vi "ViresVTD.vi"(10 "Parameters":variant, 11 "Process":refnum<class "Process.lvclass">) -> ()   [LabVIEW 2020, in "Vires VTD Engine.lvlib"]
uses:
  Vires VTD Engine.lvlib
  <vilib>/NI/NIVS Inline Async API/_VS Inline Async API/Process/Process.lvclass
  Type/Status_Cluster.ctl
  Type/ConnectionStatus.ctl
  Type/CaseSelection.ctl
  Shared/Compiled.Settings.ctl
  System Explorer/RDB Data.ctl
  RDB/RDB Object.ctl
  RDB/RDB Player Object.ctl
  Shared/Network Settings.ctl
  Shared/Protocol.ctl
  Shared/SensorInfos.ctl
  Shared/SensorInfo.ctl
  Shared/Sensor Name.ctl
  MM/MM Data.ctl
  MM/MM Objects.ctl
  MM/MM Object.ctl
  <vilib>/NI/NIVS Inline Async API/_VS Inline Async API/Process/Process.lvclass/Process.ctl
  <vilib>/NI/NIVS Inline Async API/_Data Access Engine/Access Type Classes/Write/Write.lvclass/Write.ctl
  <vilib>/NI/NIVS Inline Async API/_Data Access Engine/Access Type Classes/Read/Read.lvclass/Read.ctl
  <vilib>/NI/NIVS Inline Async API/_Data Access Engine/Data Access Engine/Methods/Write.Data.vi
  <vilib>/NI/NIVS Inline Async API/_Data Access Engine/Data Access Engine/Methods/Read.Data.vi
  <vilib>/NI/NIVS Inline Async API/_VS Inline Async API/Process/Data Member Access/Read Data Access.vi
  <vilib>/NI/NIVS Inline Async API/_VS Inline Async API/Error Handling Process/SubVIs/Error.ConvertArray.vi
  <vilib>/NI/NIVS Inline Async API/_Data Access Engine/Access Type Classes/Write/Write.ProcessData.vi
  <vilib>/NI/NIVS Inline Async API/_Data Access Engine/Access Type Classes/Read/Read.ProcessData.vi
  <vilib>/NI/NIVS Inline Async API/_Data Access Engine/Access Type Classes/Write/Write.Buffer.vi
  <vilib>/NI/NIVS Inline Async API/_Data Access Engine/Access Type Classes/Write/Write.Commit.vi
  <vilib>/NI/NIVS Inline Async API/_Data Access Engine/Data Access Engine/Methods/ReadWrite.Lookup.vi
  <vilib>/NI/NIVS Inline Async API/_Data Access Engine/Data Access Engine/Methods/Write.Lookup.vi
  <vilib>/NI/NIVS Inline Async API/_Data Access Engine/Data Access Engine/Methods/Read.Lookup.vi
  <vilib>/NI/NIVS Inline Async API/_Data Access Engine/Data Access Engine/Data Access Engine.lvclass
  RDB/RDB.lvlib
  Shared/Vires VTD Shared.lvlib
  MM/MM.lvlib
  SCP/SCP.lvlib
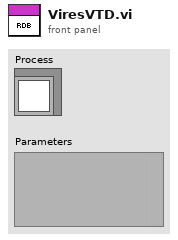
[diagram p1: front panel]
types:
  T1 = typedef "Vires VTD Engine.lvlib/Status_Cluster.ctl" = cluster{"simTime":dbl, "simFrame":dbl, "Connection Status":T2, "Connection Command":enum16{"Disconnect", "Connect"}, "Last Error":i32, "Case selection":T3}
  T2 = typedef "Vires VTD Engine.lvlib/ConnectionStatus.ctl" = enum16{"Disconnected", "Connected"}
  T3 = typedef "Vires VTD Engine.lvlib/CaseSelection.ctl" = enum32{"Idle", "Connecting", "Disconnecting", "Read/Write"}
  T4 = typedef "Vires VTD Shared.lvlib/Compiled.Settings.ctl" = cluster{"Name":string, "RDB Data Receive ":T5, "RDB Data Sent":T5, "vclient":path, "Network Settings":T8, "SensorInfos":T10, "mmanager":path, "Scenario Paths":string[], "Custom SCP Commands":string[]}
  T5 = typedef "Vires VTD Shared.lvlib/RDB Data.ctl" = T6[]
  T6 = typedef "RDB.lvlib/RDB Object.ctl" = cluster{"pkID":i32, "RDB Player Objects":T7[]}
  T7 = typedef "RDB.lvlib/RDB Player Object.ctl" = cluster{"PlayerID":i32, "Signals":string[], "WheelID":i32}
  T8 = typedef "Vires VTD Shared.lvlib/Network Settings.ctl" = cluster{"IP adress":string, "RDB":cluster{"Protocol":T9, "Tx Port":u16, "Rx Port":u16, "Buffer Size":i32, "Timeout":u16}, "SCP":cluster{"Protocol":T9, "Tx Port":u16, "Rx Port":u16, "Buffer Size":i32, "Timeout":u16}}
  T9 = typedef "Vires VTD Shared.lvlib/Protocol.ctl" = enum16{"UDP", "TCP"}
  T10 = typedef "Vires VTD Shared.lvlib/SensorInfos.ctl" = T11[]
  T11 = typedef "Vires VTD Shared.lvlib/SensorInfo.ctl" = cluster{"Sensor Name":T12, "Protocol":T9, "Network port":i32, "# Culled Objects":i32, "PlayerID":u8, "MM Data":T13}
  T12 = typedef "Vires VTD Shared.lvlib/Sensor Name.ctl" = string
  T13 = typedef "Vires VTD Shared.lvlib/MM Data.ctl" = T14[]
  T14 = typedef "MM.lvlib/MM Objects.ctl" = cluster{"pkID":i32, "MM Objects":T15[]}
  T15 = typedef "MM.lvlib/MM Object.ctl" = cluster{"Object":i32, "Signals":string[]}
  T16 = typedef "Data Access Engine.lvlib/Data Access Engine.lvclass/ReadWrite.DVR.ctl" = refnum<data-value>
  T17 = typedef "Data Access Engine.lvlib/Data Access Engine.lvclass/Write.DVR.ctl" = refnum<data-value>
  T18 = typedef "Data Access Engine.lvlib/Data Access Engine.lvclass/Read.DVR.ctl" = refnum<data-value>
  T19 = typedef "RDB.lvlib/RDB References.ctl" = cluster{"RDB Receive Reference":T20, "RDB Send Reference":T20}
  T20 = typedef "RDB.lvlib/RDB Reference.ctl" = cluster{"Conversion References":refnum<k21>[], "RDB Data":T21[], "RDB Signals":dbl[], "noSignals":i32[]}
  T21 = typedef "XNET Frame FlexRay.ctl" = cluster{"timestamp":timestamp, "payload":u8[], "slot":u16, "type":T22, "cycle count":u8, "startup?":bool, "sync?":bool, "preamble?":bool, "ch A":bool, "ch B":bool, "echo?":bool}
  T22 = typedef "XNET Frame Type FlexRay.ctl" = u8
  T23 = typedef "Vires VTD Engine.lvlib/Settings.ctl" = cluster{"UDP Receiver":refnum<k16>, "UDP Sender":refnum<k16>, "Valid Packet":bool, "TCP":refnum<k5>, "Network Settings":T8, "vclient":path}
  T24 = typedef "SCP.lvlib/SCP_Cluster.ctl" = cluster{"SCP Command ":i32, "Custom SCP Command Index":i32, "Simulation Time":i32, "Step Size":i32, "Scenario Selection":i32, "Last SCP Error":i32, "Scenario Paths":string[], "Custom SCP Commands":string[]}
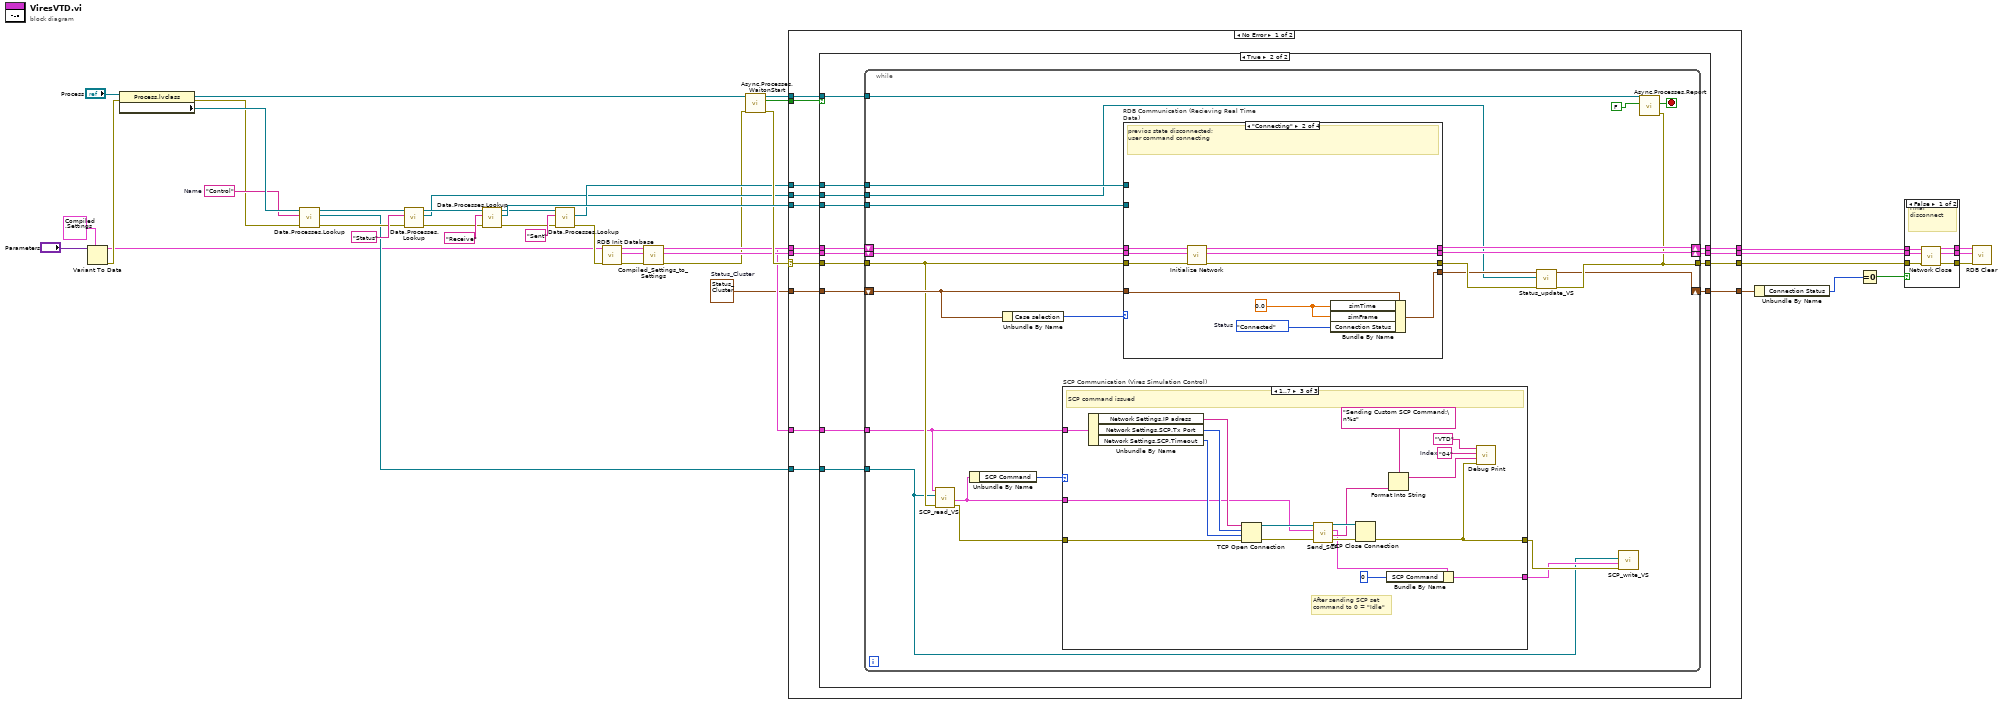
[diagram p0: block diagram]
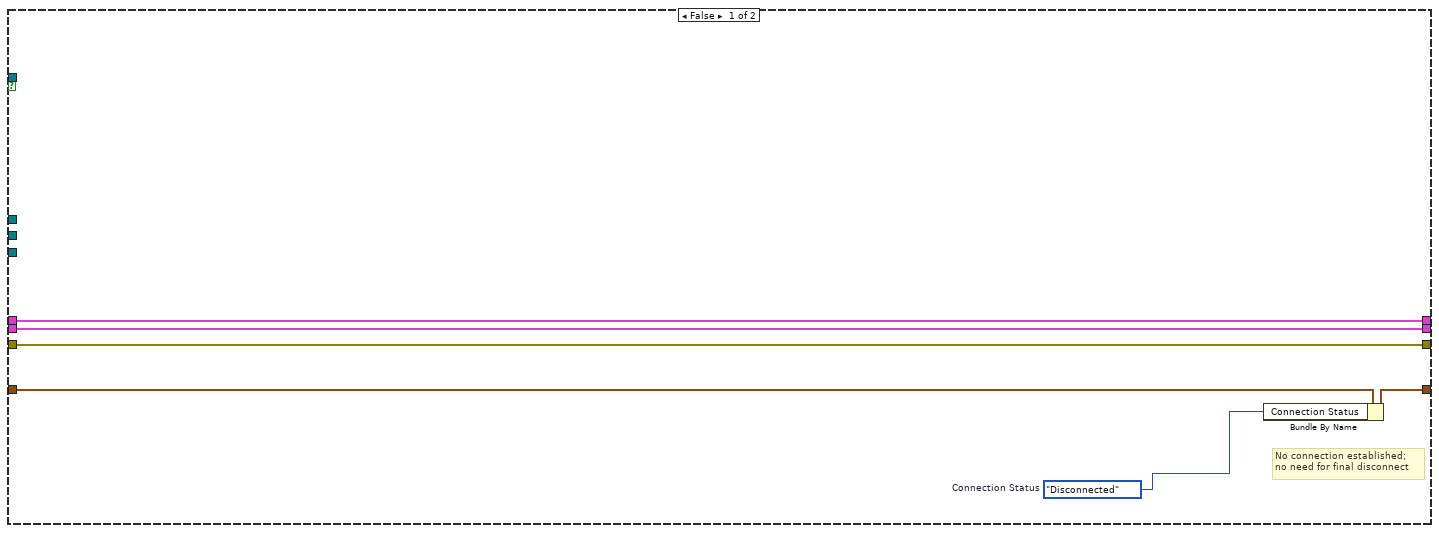
[diagram p2: hidden frame]
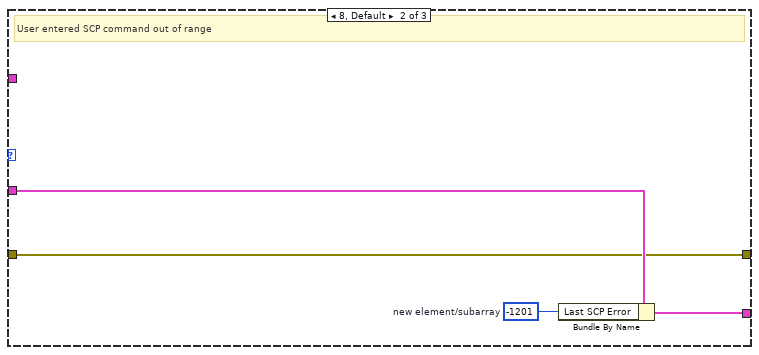
[diagram p4: hidden frame]
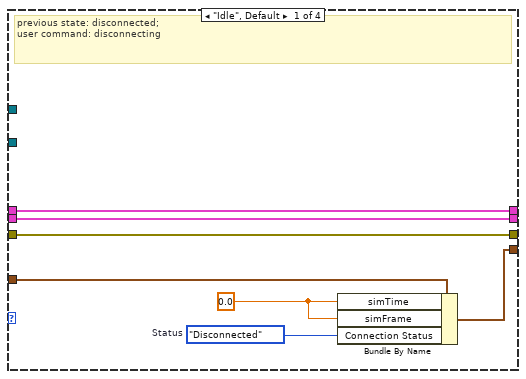
[diagram p5: hidden frame]
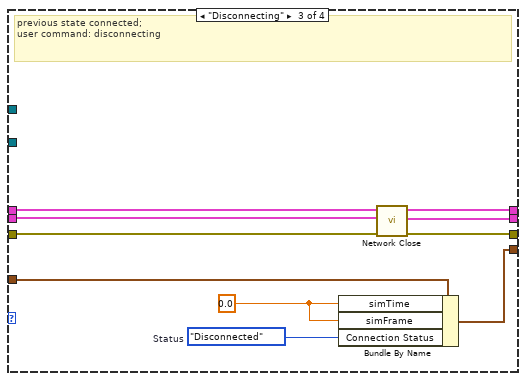
[diagram p6: hidden frame]
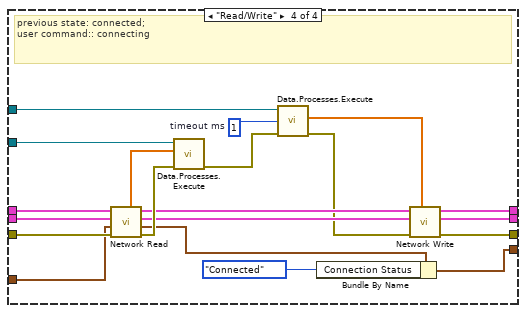
[diagram p7: hidden frame]
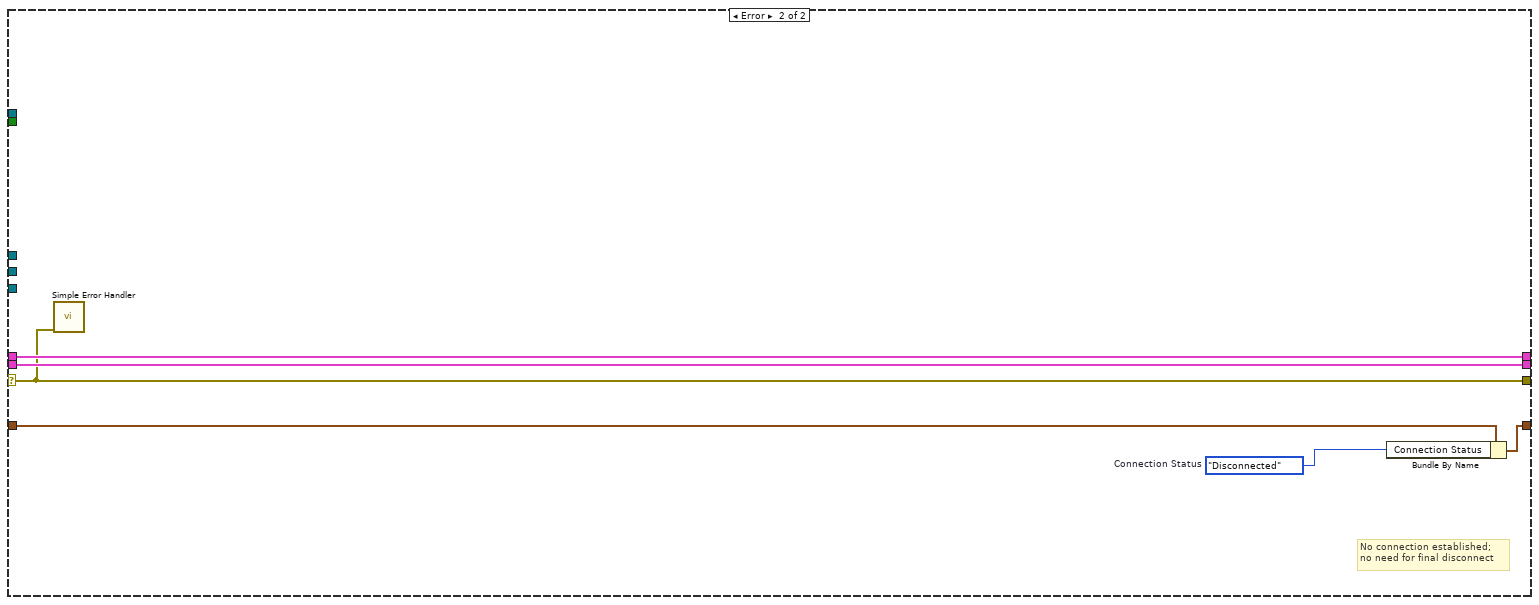
[diagram p8: hidden frame]
diagram:
  w1 = T1 {"simTime"=0.0, "simFrame"=0.0, "Connection Status"=enum."Disconnected", "Connection Command"=enum."Disconnect", "Last Error"=0, "Case selection"=enum."Connecting"}  # Status_Cluster
  w9 = "Control"  # Name
  n1 = Variant To Data(type=T4 {"Name"="", "RDB Data Receive "=[], "RDB Data Sent"=[], "vclient"=path "", "Network Settings"={"IP adress"="127.0.0.1", "RDB"={"Protocol"=enum."TCP", "Tx Port"=10, "Rx Port"=10, "Buffer Size"=204800, "Timeout"=10}, "SCP"={"Protocol"=enum."UDP", "Tx Port"=48190, "Rx Port"=48190, "Buffer Size"=204800, "Timeout"=10}}, "SensorInfos"=[], "mmanager"=path "", "Scenario Paths"=[], "Custom SCP Commands"=[]} ("Compiled.Settings"), Variant="Parameters") -> (data=w6:T4, error out=w24:errorcluster)  [unwired: 1 in]
  n2 = property class="Process.lvclass"(reference="Process", error in=w24) -> (reference out=w33:refnum<class "Process.lvclass">, error out=w7:errorcluster, "Data Member Access:Data Access"=w12:refnum<class "Data Access Engine.lvclass">)
  n3 = call-poly <vilib>:"Data.Processes.Lookup.vi"("error in (no error)"=w7, "Name"=w9, "Data Access API in"=w12) -> ("error out"=w10:errorcluster, "Ref"=w8:T16, "Data Access API out"=w11:refnum<class "Data Access Engine.lvclass">)  [unwired: 5 in, 1 out]
  n4 = call-poly <vilib>:"Data.Processes.Lookup.vi"("error in (no error)"=w10, "Name"="Status" ("Item Name"), "Data Access API in"=w11) -> ("error out"=w28:errorcluster, "Ref"=w25:T16, "Data Access API out"=w27:refnum<class "Data Access Engine.lvclass">)  [unwired: 5 in, 1 out]
  n5 = call-poly <vilib>:"Data.Processes.Lookup.vi"("error in (no error)"=w28, "Name"="Receive", "Data Access API in"=w27) -> ("error out"=w37:errorcluster, "Ref"=w36:T17, "Data Access API out"=w35:refnum<class "Data Access Engine.lvclass">)  [unwired: 5 in, 1 out]
  n6 = call-poly <vilib>:"Data.Processes.Lookup.vi"("error in (no error)"=w37, "Name"="Sent", "Data Access API in"=w35) -> ("error out"=w23:errorcluster, "Ref"=w29:T18)  [unwired: 5 in, 2 out]
  n7 = call "RDB Init Database.vi"("error in"=w23, "Compiled.Settings"=w6) -> ("error out"=w22:errorcluster, "RDB References"=w20:T19, "Compiled.Settings"=w4:T4)  [unwired: 7 in]
  n8 = call "Compiled_Settings_to_Settings.vi"("error in (no error)"=w22, "Compiled.Settings"=w4) -> ("error out"=w5:errorcluster, "Settings"=w21:T23)  [unwired: 8 in]
  n9 = call <vilib>:"Async.Processes.WaitonStart.vi"("error in (no error)"=w5, "Process"=w33) -> ("error out"=w31:errorcluster, "Execute"=w41:bool, "Process out"=w40:refnum<class "Process.lvclass">)  [unwired: 7 in]
  n10 = case shown="No Error" w31 {
    selector: w31 -> [w51 w176]
    tunnel: w41 -> [w56 _]
    tunnel: w40 -> [w55 _]
    tunnel: w36 -> [w54 _]
    tunnel: w21 -> [w53 w178]
    tunnel: w20 -> [w52 w177]
    tunnel: w29 -> [w50 _]
    tunnel: [w49 w178] -> w15
    tunnel: [w48 w177] -> w14
    tunnel: w25 -> [w47 _]
    tunnel: [w46 w176] -> w16
    tunnel: w8 -> [w45 _]
    tunnel: w4 -> [w44 _]
    tunnel: [w43 w175] -> w3
    tunnel: w1 -> [w42 w174]
    frame No Error {
      n11 = case shown="True" w56 {
        tunnel: w51 -> [w60 w67]
        tunnel: w55 -> [_ w69]
        tunnel: w54 -> [_ w76]
        tunnel: w53 -> [w62 w68]
        tunnel: w52 -> [w61 w75]
        tunnel: w50 -> [_ w74]
        tunnel: [w62 w73] -> w49
        tunnel: [w61 w72] -> w48
        tunnel: w47 -> [_ w71]
        tunnel: [w60 w70] -> w46
        tunnel: w45 -> [_ w66]
        tunnel: w44 -> [_ w65]
        tunnel: [w59 w64] -> w43
        tunnel: w42 -> [w58 w63]
        frame False {
          w57 = ConnectionStatus."Disconnected"  # Connection Status
          # "No connection established;\nno need for final disconnect"
          n12 = Bundle By Name(cluster=w58, "Connection Status"=w57) -> (w59:T1)
        }
        frame True {
          n13 = while {
            tunnel: w69 -> [w100]
            tunnel: w76 -> [w98]
            shift-right: [w94] -> w72
            shift-left: w75 -> [w97]
            tunnel: w74 -> [w95]
            shift-right: [w93] -> w73
            shift-left: w68 -> [w92]
            tunnel: w71 -> [w84]
            tunnel: w67 -> [w80]
            tunnel: [w87] -> w70
            tunnel: w66 -> [w78]
            tunnel: w65 -> [w77]
            shift-right: [w86] -> w64
            shift-left: w63 -> [w89]
            stop <- w99 stop-if-true
            # "RDB Communication"
            n14 = call "SCP_read_VS.vi"("error_in"=w80, "Ref"=w78, "Compiled.Settings"=w77) -> ("error_out"=w79:errorcluster, "SCP_Cluster_out"=w81:T24)  [unwired: 7 in]
            n15 = Unbundle By Name(w81) -> ("SCP Command"=w91:i32)
            n16 = Unbundle By Name(w89) -> ("Case selection"=w90:T3)
            n17 = case "SCP Communication (Vires Simulation Control)" shown="1..7" w91 {
              tunnel: [w101 w103 w113] -> w83
              tunnel: w79 -> [w101 w103 w112]
              tunnel: w77 -> [_ _ w111]
              tunnel: w81 -> [w102 w106 w110]
              tunnel: [w102 w104 w107] -> w82
              frame 0 {
                # "no SCP command issued;\nupdate VS UI"
              }
              frame 8, Default {
                w105 = -1201  # new element/subarray
                # "User entered SCP command out of range"
                n18 = Bundle By Name(cluster=w106, "Last SCP Error"=w105) -> (w104:T24)
              }
              frame 1..7 {
                w118 = "04"  # Index
                # "After sending SCP set\ncommand to 0 = \"Idle\""
                # "SCP command issued"
                n19 = Unbundle By Name(w111) -> ("Network Settings.IP adress"=w124:string, "Network Settings.SCP.Tx Port"=w123:u16, "Network Settings.SCP.Timeout"=w122:u16)
                n20 = TCP Open Connection(address=w124, remote port or service name=w123, timeout ms (60000)=w122, error in (no error)=w112) -> (connection ID=w121:refnum<k5>, error out=w125:errorcluster)  [unwired: 1 in]
                n21 = call "Send_SCP.vi"("error in (no error)"=w125, "SCP_Cluster_In"=w110, "TCP Network Connection in"=w121) -> ("error out"=w120:errorcluster, "CMD Msg"=w114:string, "SCP_Cluster_Out"=w109:T24, "TCP Network Connection out"=w119:refnum<k5>)  [unwired: 5 in]
                n22 = TCP Close Connection(connection ID=w119, error in (no error)=w120) -> (error out=w113:errorcluster)  [unwired: 1 in, 1 out]
                n23 = Bundle By Name(cluster=w109, "SCP Command"=0) -> (w107:T24)
                n24 = Format Into String(format string="Sending Custom SCP Command:\n%s", w114) -> (resulting string=w115:string)  [unwired: 2 in, 1 out]
                n25 = call "Debug Print.vi"("error out"=w113, "comment"=w115, "Index"=w118, "Module"="VTD") -> ()  [unwired: 8 in]
              }
            }
            n26 = case "RDB Communication (Recieving Real Time Data)" shown="\"Connecting\"" w90 {
              tunnel: w98 -> [_ _ _ w172]
              tunnel: w92 -> [w132 w141 w149 w171]
              tunnel: w97 -> [w131 w140 w148 w170]
              tunnel: w80 -> [w130 w142 w147 w169]
              tunnel: w95 -> [_ _ _ w168]
              tunnel: [w131 w138 w151 w167] -> w94
              tunnel: [w132 w139 w152 w166] -> w93
              tunnel: [w130 w137 w150 w165] -> w88
              tunnel: w89 -> [w129 w134 w144 w156]
              tunnel: [w126 w133 w143 w153] -> w85
              frame "Idle", Default {
                w128 = 0.0
                w127 = ConnectionStatus."Disconnected"  # Status
                # "previous state: disconnected; \nuser command: disconnecting"
                n27 = Bundle By Name(cluster=w129, "simTime"=w128, "simFrame"=w128, "Connection Status"=w127) -> (w126:T1)
              }
              frame "Connecting" {
                w136 = 0.0
                w135 = ConnectionStatus."Connected"  # Status
                # "previos state disconnected; \nuser command connecting"
                n28 = call "Initialize Network.vi"("error in (no error)"=w142, "RDB References"=w140, "Settings"=w141) -> ("error out"=w137:errorcluster, "RDB References"=w138:T19, "Settings"=w139:T23)  [unwired: 6 in]
                n29 = Bundle By Name(cluster=w134, "simTime"=w136, "simFrame"=w136, "Connection Status"=w135) -> (w133:T1)
              }
              frame "Disconnecting" {
                w146 = 0.0
                w145 = ConnectionStatus."Disconnected"  # Status
                # "previous state connected; \nuser command: disconnecting"
                n30 = Bundle By Name(cluster=w144, "simTime"=w146, "simFrame"=w146, "Connection Status"=w145) -> (w143:T1)
                n31 = call "Network Close.vi"("error in (no error)"=w147, "RDB References"=w148, "Settings"=w149) -> ("error out"=w150:errorcluster, "RDB References"=w151:T19, "Settings"=w152:T23)  [unwired: 6 in]
              }
              frame "Read/Write" {
                w162 = 1  # timeout ms
                # "previous state: connected; \nuser command:: connecting"
                n32 = call "Network Read.vi"("error in (no error)"=w169, "Status_Cluster_in"=w156, "RDB References in"=w170, "Settings"=w171) -> ("error out"=w164:errorcluster, "Status_Cluster_out"=w155:T1, "RDB References out"=w159:T19, "Settings"=w161:T23, "RDB Receive Reference.RDB Signals"=w163:dbl[])  [unwired: 2 in, 1 out]
                n33 = call-poly <vilib>:"Data.Processes.Execute.vi"("error in (no error)"=w164, "Values"=w163, "Ref"=w172) -> ("error out"=w157:errorcluster)  [unwired: 8 in]
                n34 = call-poly <vilib>:"Data.Processes.Execute.vi"("error in (no error)"=w157, "timeout ms"=w162, "Ref"=w168) -> ("error out"=w158:errorcluster, "Values"=w160:dbl[])  [unwired: 6 in, 1 out]
                n35 = Bundle By Name(cluster=w155, "Connection Status"=ConnectionStatus."Connected") -> (w153:T1)
                n36 = call "Network Write.vi"("Values"=w160, "error in (no error)"=w158, "RDB References in"=w159, "Settings"=w161) -> ("error out"=w165:errorcluster, "RDB Reference out"=w167:T19, "Settings"=w166:T23)  [unwired: 5 in]
              }
            }
            n37 = call "Status_update_VS.vi"("error in (no error)"=w88, "Data Value Reference in"=w84, "Status_Cluster_out in"=w85) -> ("error out"=w87:errorcluster, "Status_Cluster_out out"=w86:T1)  [unwired: 7 in]
            n38 = call "SCP_write_VS.vi"("error_in"=w83, "SCP_Cluster_in"=w82, "Ref"=w78) -> ()  [unwired: 7 in, 2 out]
            n39 = call <vilib>:"Async.Processes.Report.vi"("Error"=w87, "Stop Async on Error?"=FALSE, "Process in"=w100) -> ("Stop"=w99:bool)  [unwired: 7 in, 1 out]
          }
        }
      }
    }
    frame Error {
      w173 = ConnectionStatus."Disconnected"  # Connection Status
      # "No connection established;\nno need for final disconnect"
      n40 = call <vilib>:"Simple Error Handler.vi"("error in (no error)"=w176) -> ()  [unwired: 4 in, 5 out]
      n41 = Bundle By Name(cluster=w174, "Connection Status"=w173) -> (w175:T1)
    }
  }
  n42 = Unbundle By Name(w3) -> ("Connection Status"=w2:T2)
  n43 = Equal To 0?(x=w2) -> (x = 0?=w13:bool)
  n44 = case shown="False" w13 {
    tunnel: [w184 w187] -> w19
    tunnel: [w183 w186] -> w18
    tunnel: [w182 w185] -> w17
    tunnel: w16 -> [w181 w185]
    tunnel: w15 -> [w180 w187]
    tunnel: w14 -> [w179 w186]
    frame False {
      # "Final disconnect"
      n45 = call "Network Close.vi"("error in (no error)"=w181, "RDB References"=w179, "Settings"=w180) -> ("error out"=w182:errorcluster, "RDB References"=w183:T19, "Settings"=w184:T23)  [unwired: 6 in]
    }
    frame True {
      # "Already disconnected"
    }
  }
  n46 = call "RDB Clear.vi"("error in (no error)"=w17, "RDB References"=w18, "Settings"=w19) -> ()  [unwired: 8 in, 1 out]
